vi "MOCVD_FrontPanel.vi"() -> ()   [LabVIEW 2011]
uses:
  low_level_proc/globals.vi
  editor_lib/Flow_Globals.vi
panel:
  out "Temp Actual":dbl caption="Actual (C)" format="%.2f"
  in  "Set":bool
  in  "Temp Setpoint":dbl caption="Setpoint (C)"
  in  "Heater":bool
  in  "Spinner":bool
  in  "Heater/Spinner Remote":bool caption="Remote"
  in  "Vac Remote":bool
  in  "Vac Exhaust":bool
  in  "Atm Exhaust":bool
  in  "Clear All Relays":bool
  in  "Stop":bool
  in  "?":T1(tab)
  in  "display N2 or H2":bool=TRUE
  in  "H2N2 Remote":bool caption="Remote"
  in  "N2 Target Flow":dbl caption="Target" min=0.0 max=1000.0
  in  "H2 Target Flow":dbl caption="Target" min=0.0 max=1000.0
  out "H2N2 Actual Flow":dbl caption="Actual"
  in  "N2 On":bool caption="On"
  in  "H2 On":bool caption="On"
  in  "Al Target Flow":dbl caption="Target" min=0.0 max=100.0 format="%.1f"
  out "Al Actual Flow":dbl caption="Actual" format="%.1f"
  in  "Al Remote":bool caption="Remote"
  in  "Al Active":bool caption="Active"
  in  "Al Bubbler In":bool caption="Bubbler In"
  in  "Al Run":bool caption="Run"
  out "Ga Flow2 label":string="Flow 2 (0-10 sscm)"
  out "Ga_Flow3_Label":string="Flow 3 (0-1000 sscm)" caption="String"
  out "Ga Actual Flow2":dbl caption="Actual" format="%.2f"
  out "Ga Actual Flow1":dbl caption="Actual" format="%.2f"
  out "Ga Actual Flow3":dbl caption="Actual"
  in  "Ga Target Flow 2":dbl caption="Target" min=0.0 max=10.0 format="%.2f"
  in  "Ga Target Flow 1":dbl caption="Target" min=0.0 max=1.0 format="%.2f"
  in  "Ga Active":bool caption="Active"
  in  "Ga Bubbler In":bool caption="Bubbler In"
  in  "Ga Run":bool caption="Run"
  in  "Ga H2 Dilute":bool caption="Dilute"
  in  "Ga Remote":bool caption="Remote"
  in  "Ga Target Flow 3":dbl caption="Target" min=0.0 max=1000.0
  in  "In Target Flow":dbl caption="Target" min=0.0 max=100.0 format="%.1f"
  out "In Actual Flow":dbl caption="Actual" format="%.1f"
  in  "In Remote":bool caption="Remote"
  in  "In Active":bool caption="Active"
  in  "In Bubbler In":bool caption="Bubbler In"
  in  "In Run":bool caption="Run"
  in  "P_gas Target Flow":dbl caption="Target" min=0.0 max=1000.0 format="%.1f"
  out "P Actual Flow":dbl caption="Actual" format="%.1f"
  in  "P gas Remote":bool caption="Remote"
  in  "P gas Active":bool caption="Active"
  in  "P Gas In":bool caption="Gas In"
  in  "P gas Run":bool caption="Run"
  in  "P gas H2 Purge":bool caption="H2 Purge"
  in  "AsH3 gas Target Flow":dbl caption="Target" min=0.0 max=1000.0 format="%.2f"
  out "As Actual Flow":dbl caption="Actual" format="%.2f"
  in  "As gas Run":bool caption="Run"
  in  "As gas H2 Purge":bool caption="H2 Purge"
  in  "As gas Active":bool caption="Active"
  in  "As Gas In":bool caption="Gas In"
  in  "As gas Remote":bool caption="Remote"
  in  "Pbub Target Flow":dbl caption="Target" min=0.0 max=100.0 format="%.1f"
  out "Pbub Actual Flow":dbl caption="Actual" format="%.1f"
  in  "Pbub Remote":bool caption="Remote"
  in  "Pbub Active":bool caption="Active"
  in  "Pbub Bubbler In":bool caption="Bubbler In"
  in  "Pbub Run":bool caption="Run"
  in  "ASL Target Flow":dbl caption="Target" min=0.0 max=100.0 format="%.1f"
  out "ASL Actual Flow":dbl caption="Actual" format="%.1f"
  in  "ASL Remote":bool caption="Remote"
  in  "ASL Active":bool caption="Active"
  in  "ASL Bubbler In":bool caption="Bubbler In"
  in  "ASL Run":bool caption="Run"
  in  "P or N":enum32{"P-Dopant", "N-Dopant"}(tab)
  out "Pdop flow 2 label":string="Flow 2 (0-100 sscm)"
  out "PDop Flow3 label":string="Flow 3 (0-1000 sscm)"
  in  "P_Dop H2 Dilute":bool caption="Dilute"
  in  "P_Dop Run":bool caption="Run"
  in  "P_Dop Bubbler":bool caption="Bubbler In"
  in  "P_Dop Active":bool caption="Active"
  in  "PDop Target Flow 1":dbl caption="Target:" min=0.0 max=100.0 format="%.1f"
  in  "PDop Target Flow  2":dbl caption="Target:" min=0.0 max=100.0 format="%.1f"
  in  "PDop Target Flow  3":dbl caption="Target:" min=0.0 max=1000.0 format="%.1f"
  in  "P_Dop Remote":bool caption="Remote"
  out "Ndop flow 2 label":string="Flow 2 (0-100 sscm)"
  out "Ndop Flow 3 label":string="Flow 3 (0-1000 sscm)"
  in  "Set N Dopant Flow Rate 1":dbl caption="Target" min=0.0 max=100.0 format="%.1f"
  in  "Set N Dopant Flow Rate 2":dbl caption="Target" min=0.0 max=100.0 format="%.1f"
  in  "Set N Dopant Flow Rate 3":dbl caption="Target" min=0.0 max=1000.0 format="%#.0f"
  in  "N_Dop Remote":bool caption="Remote"
  in  "N_Dop H2 Dilute":bool caption="Dilute"
  in  "N_Dop Run":bool caption="Run"
  in  "N_Dop Active":bool caption="Active"
  in  "N_Dop Bubbler":bool caption="Bubbler In"
  in  "6940B GPIB Address":string="23"
  # "Flow (0-1000 sccm)"
  # "N2"
  # "H2"
  # "N2"
  # "H2"
  # "Flow (0-100 sscm)"
  # "Flow 1 (0-10 sscm)"
  # "Flow (0-100 sscm)"
  # "Flow (0-100 sscm)"
  # "Flow (0-10 sscm)"
  # "Flow (0-100 sscm)"
  # "Flow (0-100 sscm)"
  # "Flow 1 (0-100 sscm)"
  # "Flow 1 (0-100 sscm)"
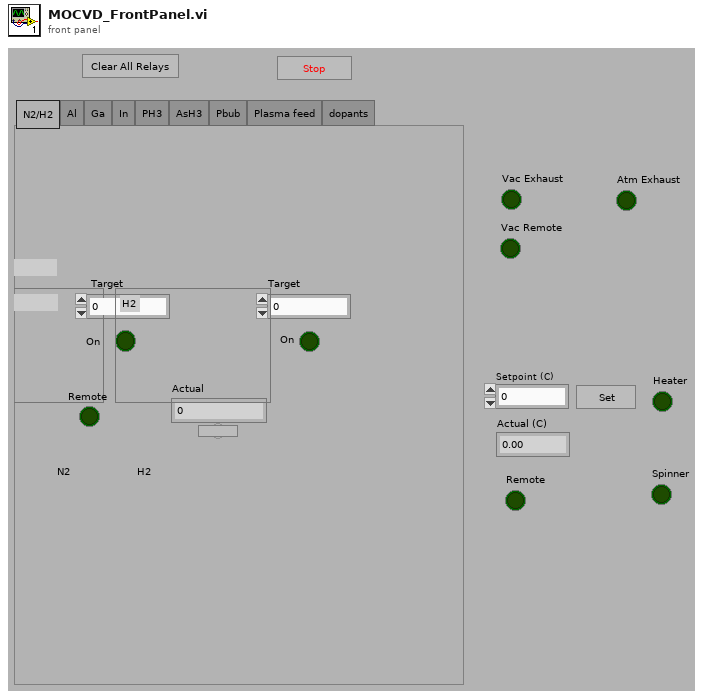
[diagram p1: front panel]
types:
  T1 = enum32{"N2/H2", "Al", "Ga", "In", "PH3", "AsH3", "Pbub", "Plasma feed", "dopants"}
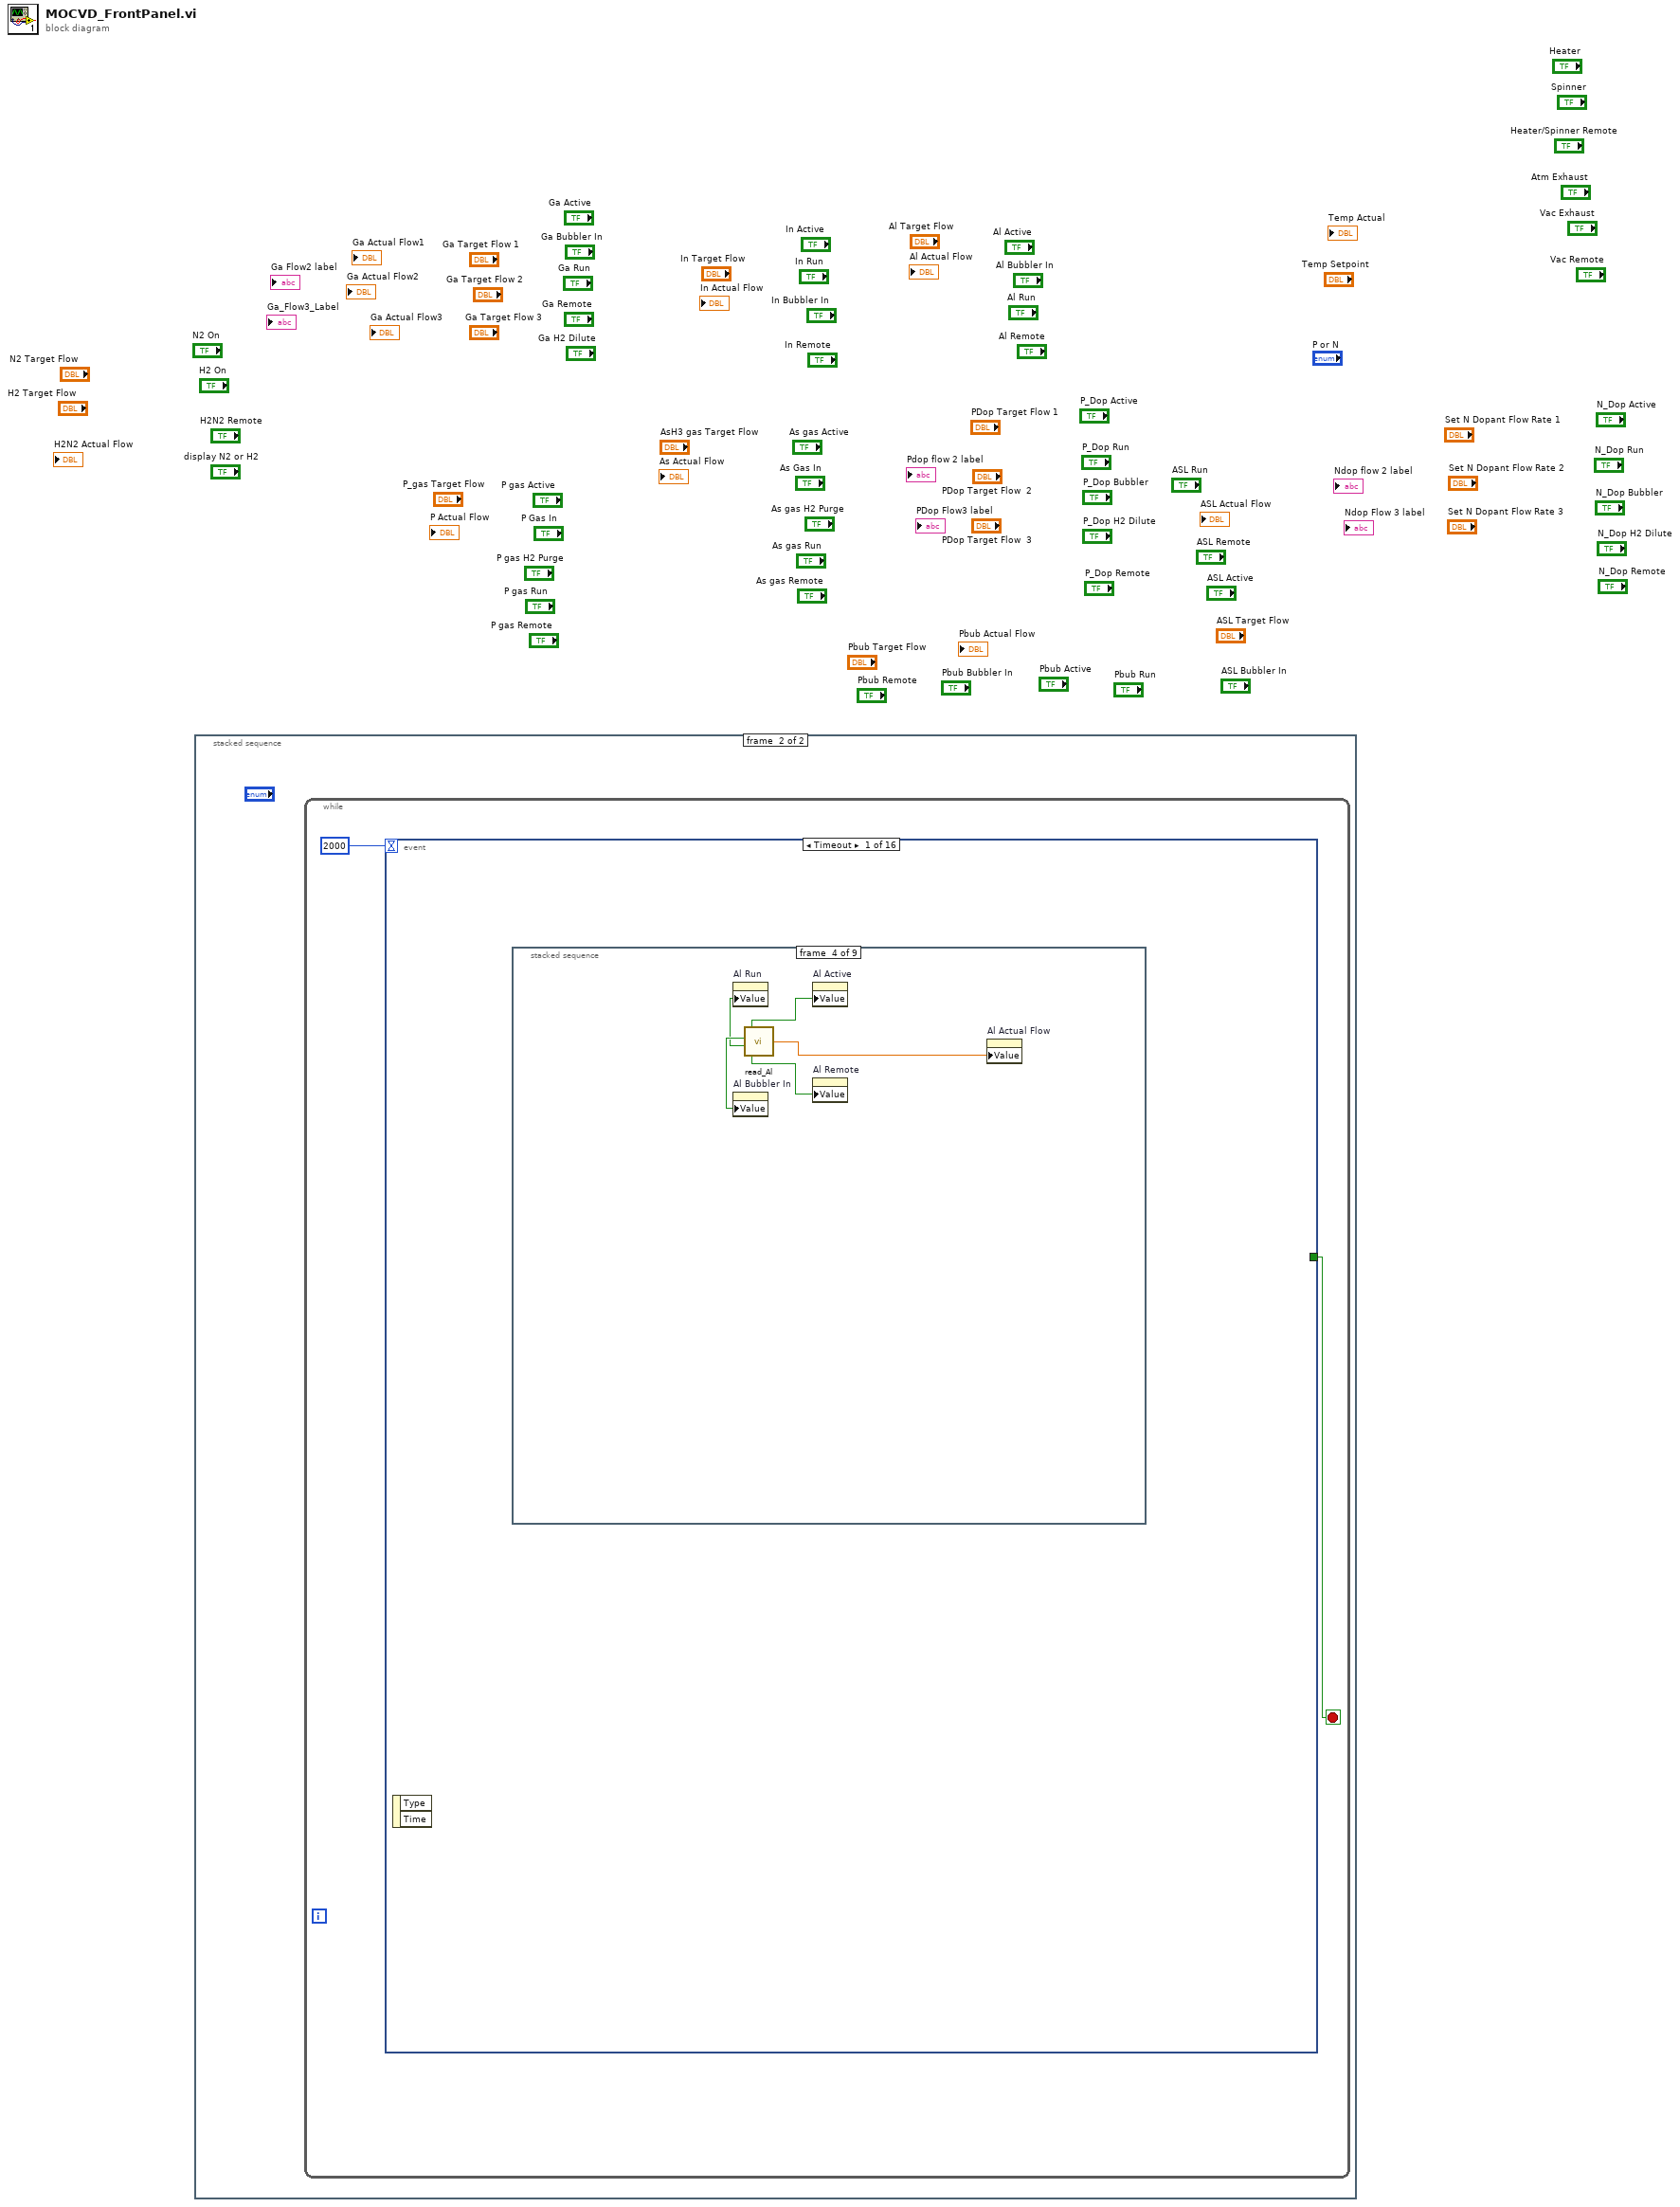
[diagram p0: block diagram]
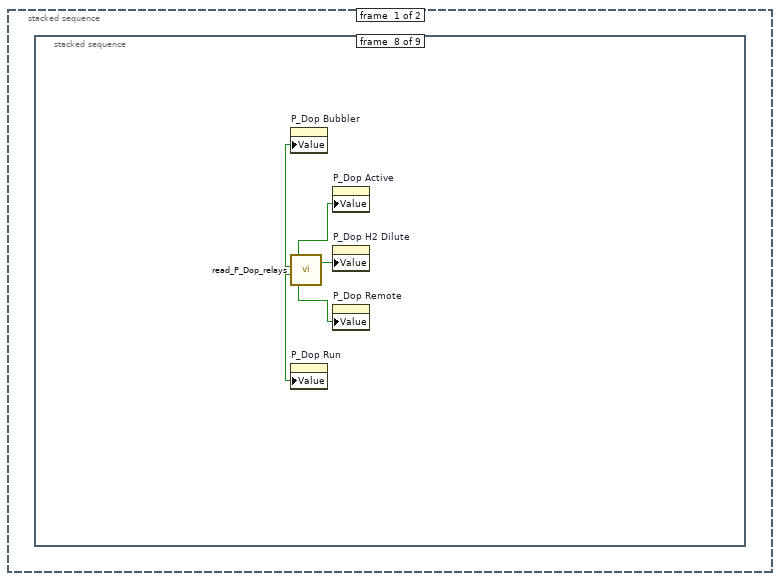
[diagram p2: hidden frame]
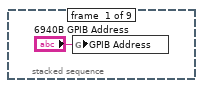
[diagram p3: hidden frame]
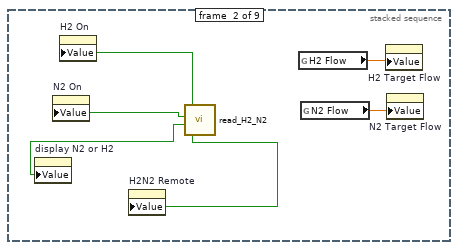
[diagram p4: hidden frame]
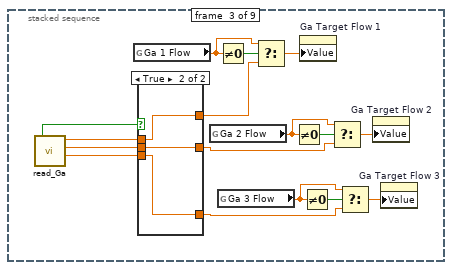
[diagram p5: hidden frame]
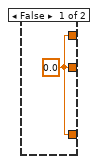
[diagram p6: hidden frame]
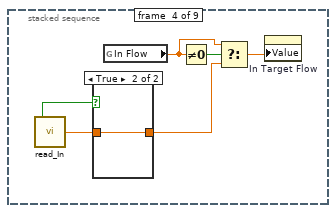
[diagram p7: hidden frame]
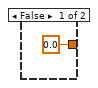
[diagram p8: hidden frame]
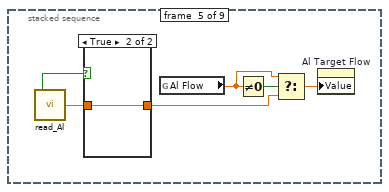
[diagram p9: hidden frame]
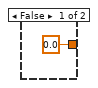
[diagram p10: hidden frame]
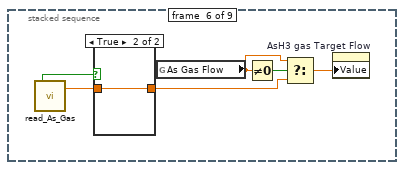
[diagram p11: hidden frame]
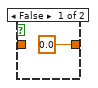
[diagram p12: hidden frame]
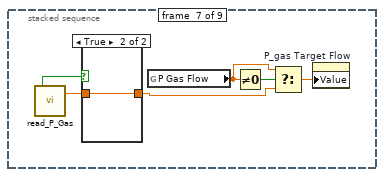
[diagram p13: hidden frame]
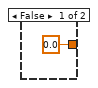
[diagram p14: hidden frame]
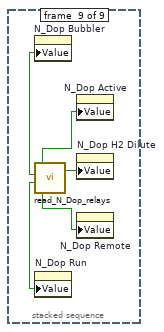
[diagram p15: hidden frame]
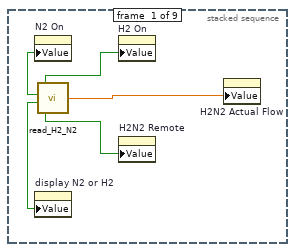
[diagram p16: hidden frame]
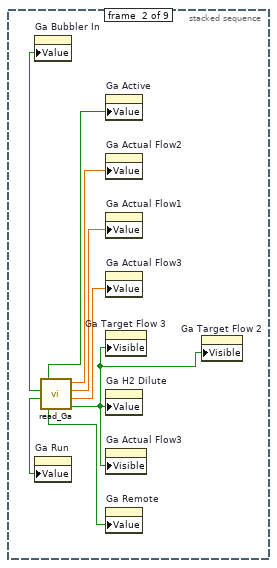
[diagram p17: hidden frame]
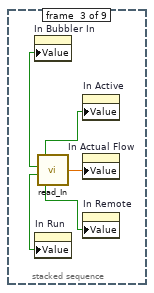
[diagram p18: hidden frame]
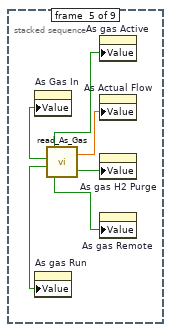
[diagram p19: hidden frame]
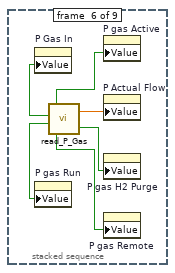
[diagram p20: hidden frame]
diagram:
  n1 = stacked-sequence {
    frame #0 {
      n2 = stacked-sequence {
        frame #0 {
          n3 = global write "globals.vi" "GPIB Address"("6940B GPIB Address") -> ()
        }
        frame #1 {
          n4 = call "read_H2_N2.vi"() -> ("Remote"=w5:bool, "Display H2N2"=w4:bool, "N2 Active"=w7:bool, "H2 Active"=w6:bool)  [unwired: 1 out]
          n5 = property on="display N2 or H2" class="Bool (strict)"("Value"=w4) -> ()  [unwired: 2 in, 2 out]
          n6 = property on="N2 On" class="Bool (strict)"("Value"=w7) -> ()  [unwired: 2 in, 2 out]
          n7 = property on="H2 On" class="Bool (strict)"("Value"=w6) -> ()  [unwired: 2 in, 2 out]
          n8 = property on="H2N2 Remote" class="Bool (strict)"("Value"=w5) -> ()  [unwired: 2 in, 2 out]
          n9 = global read "Flow_Globals.vi" "H2 Flow"() -> (w3:dbl)
          n10 = global read "Flow_Globals.vi" "N2 Flow"() -> (w2:dbl)
          n11 = property on="H2 Target Flow" class="DigNum (strict)"("Value"=w3) -> ()  [unwired: 2 in, 2 out]
          n12 = property on="N2 Target Flow" class="DigNum (strict)"("Value"=w2) -> ()  [unwired: 2 in, 2 out]
        }
        frame #2 {
          n13 = call "read_Ga.vi"() -> ("GAMFC3"=w22:dbl, "GAMFC2"=w23:dbl, "GAMFC1"=w21:dbl, "Active"=w20:bool)  [unwired: 4 out]
          n14 = global read "Flow_Globals.vi" "Ga 1 Flow"() -> (w18:dbl)
          n15 = case shown="True" w20 {
            tunnel: w23 -> [_ w26]
            tunnel: w22 -> [_ w25]
            tunnel: w21 -> [_ w27]
            tunnel: [w24 w27] -> w17
            tunnel: [w24 w26] -> w13
            tunnel: [w24 w25] -> w9
            frame False {
              w24 = 0.0 ("GAMFC2")
            }
            frame True {
            }
          }
          n16 = global read "Flow_Globals.vi" "Ga 2 Flow"() -> (w14:dbl)
          n17 = Not Equal To 0?(x=w18) -> (x != 0?=w19:bool)
          n18 = global read "Flow_Globals.vi" "Ga 3 Flow"() -> (w10:dbl)
          n19 = Select(t=w18, s=w19, f=w17) -> (s? t:f=w16:dbl)
          n20 = Not Equal To 0?(x=w14) -> (x != 0?=w15:bool)
          n21 = property on="Ga Target Flow 1" class="DigNum (strict)"("Value"=w16) -> ()  [unwired: 2 in, 2 out]
          n22 = Not Equal To 0?(x=w10) -> (x != 0?=w11:bool)
          n23 = Select(t=w14, s=w15, f=w13) -> (s? t:f=w12:dbl)
          n24 = Select(t=w10, s=w11, f=w9) -> (s? t:f=w8:dbl)
          n25 = property on="Ga Target Flow 2" class="DigNum (strict)"("Value"=w12) -> ()  [unwired: 2 in, 2 out]
          n26 = property on="Ga Target Flow 3" class="DigNum (strict)"("Value"=w8) -> ()  [unwired: 2 in, 2 out]
        }
        frame #3 {
          n27 = call "read_In.vi"() -> ("INMFC1"=w32:dbl, "Active"=w33:bool)  [unwired: 3 out]
          n28 = case shown="True" w33 {
            tunnel: [0.0 ("Actual In Flow Rate") w35] -> w29
            tunnel: w32 -> [_ w35]
            frame False {
            }
            frame True {
            }
          }
          n29 = global read "Flow_Globals.vi" "In Flow"() -> (w30:dbl)
          n30 = Not Equal To 0?(x=w30) -> (x != 0?=w31:bool)
          n31 = Select(t=w30, s=w31, f=w29) -> (s? t:f=w28:dbl)
          n32 = property on="In Target Flow" class="DigNum (strict)"("Value"=w28) -> ()  [unwired: 2 in, 2 out]
        }
        frame #4 {
          n33 = call "read_Al.vi"() -> ("ALMFC1"=w41:dbl, "Active"=w40:bool)  [unwired: 3 out]
          n34 = case shown="True" w40 {
            tunnel: [0.0 ("Actual Al Flow Rate") w43] -> w37
            tunnel: w41 -> [_ w43]
            frame False {
            }
            frame True {
            }
          }
          n35 = global read "Flow_Globals.vi" "Al Flow"() -> (w38:dbl)
          n36 = Not Equal To 0?(x=w38) -> (x != 0?=w39:bool)
          n37 = Select(t=w38, s=w39, f=w37) -> (s? t:f=w36:dbl)
          n38 = property on="Al Target Flow" class="DigNum (strict)"("Value"=w36) -> ()  [unwired: 2 in, 2 out]
        }
        frame #5 {
          n39 = call "read_As_Gas.vi"() -> ("As Gas Actual Flow Rate"=w48:dbl, "Active"=w49:bool)  [unwired: 4 out]
          n40 = case shown="True" w49 {
            tunnel: w48 -> [_ w51]
            tunnel: [0.0 ("As Gas Actual Flow Rate") w51] -> w45
            frame False {
            }
            frame True {
            }
          }
          n41 = global read "Flow_Globals.vi" "As Gas Flow"() -> (w46:dbl)
          n42 = Not Equal To 0?(x=w46) -> (x != 0?=w47:bool)
          n43 = Select(t=w46, s=w47, f=w45) -> (s? t:f=w44:dbl)
          n44 = property on="AsH3 gas Target Flow" class="DigNum (strict)"("Value"=w44) -> ()  [unwired: 2 in, 2 out]
        }
        frame #6 {
          n45 = call "read_P_Gas.vi"() -> ("P Gas Actual Flow Rate"=w56:dbl, "Active"=w57:bool)  [unwired: 4 out]
          n46 = case shown="True" w57 {
            tunnel: [0.0 ("P Gas Actual Flow Rate") w59] -> w53
            tunnel: w56 -> [_ w59]
            frame False {
            }
            frame True {
            }
          }
          n47 = global read "Flow_Globals.vi" "P Gas Flow"() -> (w54:dbl)
          n48 = Not Equal To 0?(x=w54) -> (x != 0?=w55:bool)
          n49 = Select(t=w54, s=w55, f=w53) -> (s? t:f=w52:dbl)
          n50 = property on="P_gas Target Flow" class="DigNum (strict)"("Value"=w52) -> ()  [unwired: 2 in, 2 out]
        }
        frame #7 {
          n51 = call "read_P_Dop_relays.vi"() -> ("P_Dop H2 Dilute"=w64:bool, "P_Dop Remote"=w61:bool, "P_Dop Run"=w62:bool, "P_Dop Bubbler"=w60:bool, "P_Dop Active"=w63:bool)  [unwired: 1 out]
          n52 = property on="P_Dop Bubbler" class="Bool (strict)"("Value"=w60) -> ()  [unwired: 2 in, 2 out]
          n53 = property on="P_Dop Run" class="Bool (strict)"("Value"=w62) -> ()  [unwired: 2 in, 2 out]
          n54 = property on="P_Dop Active" class="Bool (strict)"("Value"=w63) -> ()  [unwired: 2 in, 2 out]
          n55 = property on="P_Dop H2 Dilute" class="Bool (strict)"("Value"=w64) -> ()  [unwired: 2 in, 2 out]
          n56 = property on="P_Dop Remote" class="Bool (strict)"("Value"=w61) -> ()  [unwired: 2 in, 2 out]
        }
        frame #8 {
          n57 = call "read_N_Dop_relays.vi"() -> ("N_Dop H2 Dilute"=w69:bool, "N_Dop Remote"=w68:bool, "N_Dop Run"=w67:bool, "N_Dop Bubbler"=w66:bool, "N_Dop Active"=w65:bool)  [unwired: 1 out]
          n58 = property on="N_Dop Bubbler" class="Bool (strict)"("Value"=w66) -> ()  [unwired: 2 in, 2 out]
          n59 = property on="N_Dop Run" class="Bool (strict)"("Value"=w67) -> ()  [unwired: 2 in, 2 out]
          n60 = property on="N_Dop Active" class="Bool (strict)"("Value"=w65) -> ()  [unwired: 2 in, 2 out]
          n61 = property on="N_Dop H2 Dilute" class="Bool (strict)"("Value"=w69) -> ()  [unwired: 2 in, 2 out]
          n62 = property on="N_Dop Remote" class="Bool (strict)"("Value"=w68) -> ()  [unwired: 2 in, 2 out]
        }
      }
    }
    frame #1 {
      n63 = while {
        stop <- w71 stop-if-true
        n64 = event shown="[0] Timeout" {
          selector: _ -> [_ _ _ _ _ _ _ _ _ _ _ _ _ _ _ _]
          dyn-events: _ -> [_ _ _ _ _ _ _ _ _ _ _ _ _ _ _ _]
          timeout: 2000 -> [_ _ _ _ _ _ _ _ _ _ _ _ _ _ _ _]
          tunnel: [_ _ _ "Stop" _ _ _ _ _ _ _ _ _ _ _ _] -> w71
          event Timeout {
            n65 = event-data() -> ()  [unwired: 3 out]
            n66 = stacked-sequence {
              frame #0 {
                n67 = call "read_H2_N2.vi"() -> ("H2N2 Flow Rate"=w72:dbl, "Remote"=w76:bool, "Display H2N2"=w75:bool, "N2 Active"=w74:bool, "H2 Active"=w73:bool)
                n68 = property on="N2 On" class="Bool (strict)"("Value"=w74) -> ()  [unwired: 2 in, 2 out]
                n69 = property on="display N2 or H2" class="Bool (strict)"("Value"=w75) -> ()  [unwired: 2 in, 2 out]
                n70 = property on="H2 On" class="Bool (strict)"("Value"=w73) -> ()  [unwired: 2 in, 2 out]
                n71 = property on="H2N2 Remote" class="Bool (strict)"("Value"=w76) -> ()  [unwired: 2 in, 2 out]
                n72 = property on="H2N2 Actual Flow" class="DigNum (strict)"("Value"=w72) -> ()  [unwired: 2 in, 2 out]
              }
              frame #1 {
                n73 = call "read_Ga.vi"() -> ("H2 Dilute"=w77:bool, "GAMFC3"=w78:dbl, "GAMFC2"=w80:dbl, "GAMFC1"=w79:dbl, "Remote"=w83:bool, "Run"=w84:bool, "Bubbler In"=w81:bool, "Active"=w82:bool)
                n74 = property on="Ga Bubbler In" class="Bool (strict)"("Value"=w81) -> ()  [unwired: 2 in, 2 out]
                n75 = property on="Ga Run" class="Bool (strict)"("Value"=w84) -> ()  [unwired: 2 in, 2 out]
                n76 = property on="Ga Active" class="Bool (strict)"("Value"=w82) -> ()  [unwired: 2 in, 2 out]
                n77 = property on="Ga Actual Flow2" class="DigNum (strict)"("Value"=w79) -> ()  [unwired: 2 in, 2 out]
                n78 = property on="Ga Actual Flow1" class="DigNum (strict)"("Value"=w80) -> ()  [unwired: 2 in, 2 out]
                n79 = property on="Ga Actual Flow3" class="DigNum (strict)"("Value"=w78) -> ()  [unwired: 2 in, 2 out]
                n80 = property on="Ga Target Flow 3" class="DigNum (strict)"("Visible"=w77) -> ()  [unwired: 2 in, 2 out]
                n81 = property on="Ga H2 Dilute" class="Bool (strict)"("Value"=w77) -> ()  [unwired: 2 in, 2 out]
                n82 = property on="Ga Actual Flow3" class="DigNum (strict)"("Visible"=w77) -> ()  [unwired: 2 in, 2 out]
                n83 = property on="Ga Remote" class="Bool (strict)"("Value"=w83) -> ()  [unwired: 2 in, 2 out]
                n84 = property on="Ga Target Flow 2" class="DigNum (strict)"("Visible"=w77) -> ()  [unwired: 2 in, 2 out]
              }
              frame #2 {
                n85 = call "read_In.vi"() -> ("INMFC1"=w85:dbl, "Remote"=w87:bool, "Run"=w86:bool, "Bubbler In"=w88:bool, "Active"=w89:bool)
                n86 = property on="In Bubbler In" class="Bool (strict)"("Value"=w88) -> ()  [unwired: 2 in, 2 out]
                n87 = property on="In Run" class="Bool (strict)"("Value"=w86) -> ()  [unwired: 2 in, 2 out]
                n88 = property on="In Active" class="Bool (strict)"("Value"=w89) -> ()  [unwired: 2 in, 2 out]
                n89 = property on="In Actual Flow" class="DigNum (strict)"("Value"=w85) -> ()  [unwired: 2 in, 2 out]
                n90 = property on="In Remote" class="Bool (strict)"("Value"=w87) -> ()  [unwired: 2 in, 2 out]
              }
              frame #3 {
                n91 = call "read_Al.vi"() -> ("ALMFC1"=w90:dbl, "Remote"=w91:bool, "Run"=w92:bool, "Bubbler In"=w93:bool, "Active"=w94:bool)
                n92 = property on="Al Run" class="Bool (strict)"("Value"=w92) -> ()  [unwired: 2 in, 2 out]
                n93 = property on="Al Bubbler In" class="Bool (strict)"("Value"=w93) -> ()  [unwired: 2 in, 2 out]
                n94 = property on="Al Active" class="Bool (strict)"("Value"=w94) -> ()  [unwired: 2 in, 2 out]
                n95 = property on="Al Remote" class="Bool (strict)"("Value"=w91) -> ()  [unwired: 2 in, 2 out]
                n96 = property on="Al Actual Flow" class="DigNum (strict)"("Value"=w90) -> ()  [unwired: 2 in, 2 out]
              }
              frame #4 {
                n97 = call "read_As_Gas.vi"() -> ("H2 Flush"=w96:bool, "As Gas Actual Flow Rate"=w95:dbl, "Remote"=w100:bool, "Run"=w99:bool, "Gas In"=w98:bool, "Active"=w97:bool)
                n98 = property on="As Gas In" class="Bool (strict)"("Value"=w98) -> ()  [unwired: 2 in, 2 out]
                n99 = property on="As gas Run" class="Bool (strict)"("Value"=w99) -> ()  [unwired: 2 in, 2 out]
                n100 = property on="As gas Active" class="Bool (strict)"("Value"=w97) -> ()  [unwired: 2 in, 2 out]
                n101 = property on="As Actual Flow" class="DigNum (strict)"("Value"=w95) -> ()  [unwired: 2 in, 2 out]
                n102 = property on="As gas H2 Purge" class="Bool (strict)"("Value"=w96) -> ()  [unwired: 2 in, 2 out]
                n103 = property on="As gas Remote" class="Bool (strict)"("Value"=w100) -> ()  [unwired: 2 in, 2 out]
              }
              frame #5 {
                n104 = call "read_P_Gas.vi"() -> ("H2 Flush"=w102:bool, "P Gas Actual Flow Rate"=w101:dbl, "Remote"=w106:bool, "Run"=w105:bool, "Gas In"=w104:bool, "Active"=w103:bool)
                n105 = property on="P Gas In" class="Bool (strict)"("Value"=w104) -> ()  [unwired: 2 in, 2 out]
                n106 = property on="P gas Run" class="Bool (strict)"("Value"=w105) -> ()  [unwired: 2 in, 2 out]
                n107 = property on="P gas Active" class="Bool (strict)"("Value"=w103) -> ()  [unwired: 2 in, 2 out]
                n108 = property on="P Actual Flow" class="DigNum (strict)"("Value"=w101) -> ()  [unwired: 2 in, 2 out]
                n109 = property on="P gas H2 Purge" class="Bool (strict)"("Value"=w102) -> ()  [unwired: 2 in, 2 out]
                n110 = property on="P gas Remote" class="Bool (strict)"("Value"=w106) -> ()  [unwired: 2 in, 2 out]
              }
              frame #6 {
                n111 = call "read_vacuum.vi"() -> ("Vac Remote"=w109:bool, "Atm Exhaust"=w108:bool, "Vac Exhaust"=w107:bool)
                n112 = property on="Vac Exhaust" class="Bool (strict)"("Value"=w107) -> ()  [unwired: 2 in, 2 out]
                n113 = property on="Atm Exhaust" class="Bool (strict)"("Value"=w108) -> ()  [unwired: 2 in, 2 out]
                n114 = property on="Vac Remote" class="Bool (strict)"("Value"=w109) -> ()  [unwired: 2 in, 2 out]
              }
              frame #7 {
                n115 = call "read_heater_spinner.vi"() -> ("Heater/Spinner Remote"=w112:bool, "Spinner"=w111:bool, "Heater"=w110:bool)  [unwired: 7 out]
                n116 = property on="Spinner" class="Bool (strict)"("Value"=w111) -> ()  [unwired: 2 in, 2 out]
                n117 = property on="Heater/Spinner Remote" class="Bool (strict)"("Value"=w112) -> ()  [unwired: 2 in, 2 out]
                n118 = property on="Heater" class="Bool (strict)"("Value"=w110) -> ()  [unwired: 2 in, 2 out]
              }
              frame #8 {
                n119 = call "read_temp.vi"() -> ("Temperature (C)"=w113:dbl)  [unwired: 1 out]
                n120 = property on="Temp Actual" class="DigNum (strict)"("Value"=w113) -> ()  [unwired: 2 in, 2 out]
              }
            }
          }
          event "Set": Value Change {
            n121 = event-data() -> ()  [unwired: 6 out]
            n122 = property on="Temp Setpoint" class="DigNum (strict)"() -> ("Value"=w114:dbl)  [unwired: 2 in, 2 out]
            n123 = call "write_temp.vi"("Temperature (C)"=w114) -> ()  [unwired: 1 out]
          }
          event "Clear All Relays": Mouse Down {
            n124 = event-data() -> ()  [unwired: 8 out]
            n125 = flat-sequence {
              frame #0 {
                n126 = call "clear_all_relays.vi"() -> ()  [unwired: 2 out]
              }
              frame #1 {
                n127 = property on="Clear All Relays" class="Bool (strict)"("Value"=FALSE ("Clear All Relays")) -> ()  [unwired: 2 in, 2 out]
              }
            }
          }
          event "Stop": Value Change {
            n128 = event-data() -> ()  [unwired: 7 out]
          }
          event "H2N2 Remote", "display N2 or H2", "N2 On", "H2 On", "N2 Target Flow", "H2 Target Flow": Value Change {
            n129 = event-data() -> ()  [unwired: 7 out]
            n130 = property on="H2 On" class="Bool (strict)"() -> ("Value"=w118:bool)  [unwired: 2 in, 2 out]
            n131 = property on="H2 Target Flow" class="DigNum (strict)"() -> ("Value"=w121:dbl)  [unwired: 2 in, 2 out]
            n132 = property on="H2N2 Remote" class="Bool (strict)"() -> ("Value"=w117:bool)  [unwired: 2 in, 2 out]
            n133 = property on="N2 Target Flow" class="DigNum (strict)"() -> ("Value"=w120:dbl)  [unwired: 2 in, 2 out]
            n134 = property on="N2 On" class="Bool (strict)"() -> ("Value"=w119:bool)  [unwired: 2 in, 2 out]
            n135 = property on="display N2 or H2" class="Bool (strict)"() -> ("Value"=w122:bool)  [unwired: 2 in, 2 out]
            n136 = call "set_H2N2_display.vi"("Manifold N2 Flow"=w120, "Manifold H2 Flow"=w121, "Display H2 or N2"=w122, "H2 Active"=w118, "N2 Active"=w119, "Remote"=w117) -> ()
          }
          event "In Remote", "In Active", "In Bubbler In", "In Run", "In Target Flow": Value Change {
            n137 = event-data() -> ()  [unwired: 7 out]
            n138 = property on="In Target Flow" class="DigNum (strict)"() -> ("Value"=w127:dbl)  [unwired: 2 in, 2 out]
            n139 = property on="In Bubbler In" class="Bool (strict)"() -> ("Value"=w123:bool)  [unwired: 2 in, 2 out]
            n140 = property on="In Run" class="Bool (strict)"() -> ("Value"=w125:bool)  [unwired: 2 in, 2 out]
            n141 = property on="In Active" class="Bool (strict)"() -> ("Value"=w124:bool)  [unwired: 2 in, 2 out]
            n142 = property on="In Remote" class="Bool (strict)"() -> ("Value"=w126:bool)  [unwired: 2 in, 2 out]
            n143 = call "set_In.vi"("INMFC1"=w127, "Remote"=w126, "Run"=w125, "Bubbler In"=w123, "Active"=w124) -> ()  [unwired: 5 in]
          }
          event "Pbub Remote", "Pbub Active", "Pbub Bubbler In", "Pbub Run", "Pbub Target Flow": Value Change {
            n144 = event-data() -> ()  [unwired: 7 out]
            n145 = property on="Pbub Target Flow" class="DigNum (strict)"() -> ("Value"=w132:dbl)  [unwired: 2 in, 2 out]
            n146 = property on="Pbub Run" class="Bool (strict)"() -> ("Value"=w129:bool)  [unwired: 2 in, 2 out]
            n147 = property on="Pbub Bubbler In" class="Bool (strict)"() -> ("Value"=w130:bool)  [unwired: 2 in, 2 out]
            n148 = property on="Pbub Active" class="Bool (strict)"() -> ("Value"=w131:bool)  [unwired: 2 in, 2 out]
            n149 = property on="Pbub Remote" class="Bool (strict)"() -> ("Value"=w128:bool)  [unwired: 2 in, 2 out]
            n150 = call "set_P_Liq.vi"("flow 1"=w132, "Remote"=w128, "Run"=w129, "Bubbler In"=w130, "Active"=w131) -> ()  [unwired: 5 in]
          }
          event "ASL Target Flow", "ASL Active", "ASL Bubbler In", "ASL Run", "ASL Remote": Value Change {
            n151 = event-data() -> ()  [unwired: 7 out]
            n152 = property on="ASL Active" class="Bool (strict)"() -> ("Value"=w136:bool)  [unwired: 2 in, 2 out]
            n153 = property on="ASL Bubbler In" class="Bool (strict)"() -> ("Value"=w135:bool)  [unwired: 2 in, 2 out]
            n154 = property on="ASL Run" class="Bool (strict)"() -> ("Value"=w134:bool)  [unwired: 2 in, 2 out]
            n155 = property on="ASL Target Flow" class="DigNum (strict)"() -> ("Value"=w137:dbl)  [unwired: 2 in, 2 out]
            n156 = property on="ASL Remote" class="Bool (strict)"() -> ("Value"=w133:bool)  [unwired: 2 in, 2 out]
            n157 = call "set_As_Liq.vi"("ASLMFC1"=w137, "Remote"=w133, "Run"=w134, "Bubbler In"=w135, "Active"=w136) -> ()  [unwired: 5 in]
          }
          event "Al Remote", "Al Active", "Al Bubbler In", "Al Run", "Al Target Flow": Value Change {
            n158 = event-data() -> ()  [unwired: 7 out]
            n159 = property on="Al Target Flow" class="DigNum (strict)"() -> ("Value"=w142:dbl)  [unwired: 2 in, 2 out]
            n160 = property on="Al Bubbler In" class="Bool (strict)"() -> ("Value"=w140:bool)  [unwired: 2 in, 2 out]
            n161 = property on="Al Active" class="Bool (strict)"() -> ("Value"=w141:bool)  [unwired: 2 in, 2 out]
            n162 = property on="Al Run" class="Bool (strict)"() -> ("Value"=w139:bool)  [unwired: 2 in, 2 out]
            n163 = property on="Al Remote" class="Bool (strict)"() -> ("Value"=w138:bool)  [unwired: 2 in, 2 out]
            n164 = call "set_Al.vi"("ALMFC1"=w142, "Remote"=w138, "Run"=w139, "Bubbler In"=w140, "Active"=w141) -> ()  [unwired: 5 out]
          }
          event "P gas Remote", "P gas Active", "P Gas In", "P gas Run", "P gas H2 Purge", "P_gas Target Flow": Value Change {
            n165 = event-data() -> ()  [unwired: 7 out]
            n166 = property on="P_gas Target Flow" class="DigNum (strict)"() -> ("Value"=w148:dbl)  [unwired: 2 in, 2 out]
            n167 = property on="P gas Active" class="Bool (strict)"() -> ("Value"=w147:bool)  [unwired: 2 in, 2 out]
            n168 = property on="P Gas In" class="Bool (strict)"() -> ("Value"=w146:bool)  [unwired: 2 in, 2 out]
            n169 = property on="P gas H2 Purge" class="Bool (strict)"() -> ("Value"=w145:bool)  [unwired: 2 in, 2 out]
            n170 = property on="P gas Run" class="Bool (strict)"() -> ("Value"=w144:bool)  [unwired: 2 in, 2 out]
            n171 = property on="P gas Remote" class="Bool (strict)"() -> ("Value"=w143:bool)  [unwired: 2 in, 2 out]
            n172 = call "set_P_gas.vi"("Run"=w144, "Gas In"=w146, "Active"=w147, "P_Gas Remote"=w143, "H2 Flush"=w145, "P_Gas Flow"=w148) -> ()
          }
          event "As gas Remote", "As gas Run", "As gas H2 Purge", "As Gas In", "As gas Active", "AsH3 gas Target Flow": Value Change {
            n173 = event-data() -> ()  [unwired: 7 out]
            n174 = property on="AsH3 gas Target Flow" class="DigNum (strict)"() -> ("Value"=w154:dbl)  [unwired: 2 in, 2 out]
            n175 = property on="As gas Active" class="Bool (strict)"() -> ("Value"=w153:bool)  [unwired: 2 in, 2 out]
            n176 = property on="As Gas In" class="Bool (strict)"() -> ("Value"=w152:bool)  [unwired: 2 in, 2 out]
            n177 = property on="As gas H2 Purge" class="Bool (strict)"() -> ("Value"=w151:bool)  [unwired: 2 in, 2 out]
            n178 = property on="As gas Run" class="Bool (strict)"() -> ("Value"=w150:bool)  [unwired: 2 in, 2 out]
            n179 = property on="As gas Remote" class="Bool (strict)"() -> ("Value"=w149:bool)  [unwired: 2 in, 2 out]
            n180 = call "set_As_gas.vi"("Active"=w153, "As_Gas Flow"=w154, "Gas In"=w152, "H2 Flush"=w151, "Run"=w150, "Remote"=w149) -> ()  [unwired: 10 out]
          }
          event "Ga Active", "Ga Bubbler In", "Ga Run", "Ga Target Flow 1", "Ga Target Flow 2", "Ga Target Flow 3", "Ga Remote", "Ga H2 Dilute": Value Change {
            n181 = event-data() -> ()  [unwired: 6 out]
            n182 = property on="Ga Bubbler In" class="Bool (strict)"() -> ("Value"=w159:bool)  [unwired: 2 in, 2 out]
            n183 = property on="Ga Target Flow 1" class="DigNum (strict)"() -> ("Value"=w162:dbl)  [unwired: 2 in, 2 out]
            n184 = property on="Ga Target Flow 2" class="DigNum (strict)"() -> ("Value"=w161:dbl)  [unwired: 2 in, 2 out]
            n185 = property on="Ga Target Flow 3" class="DigNum (strict)"() -> ("Value"=w160:dbl)  [unwired: 2 in, 2 out]
            n186 = property on="Ga Active" class="Bool (strict)"() -> ("Value"=w158:bool)  [unwired: 2 in, 2 out]
            n187 = property on="Ga Run" class="Bool (strict)"() -> ("Value"=w156:bool)  [unwired: 2 in, 2 out]
            n188 = property on="Ga Remote" class="Bool (strict)"() -> ("Value"=w157:bool)  [unwired: 2 in, 2 out]
            n189 = property on="Ga H2 Dilute" class="Bool (strict)"() -> ("Value"=w155:bool)  [unwired: 2 in, 2 out]
            n190 = call "set_Ga.vi"("Active"=w158, "GAMFC3"=w160, "GAMFC2"=w161, "GAMFC1"=w162, "Bubbler In"=w159, "H2 Dilute"=w155, "Run"=w156, "Remote"=w157) -> ()  [unwired: 8 out]
            n191 = property on="Ga Actual Flow3" class="DigNum (strict)"("Visible"=w155) -> ()  [unwired: 2 in, 2 out]
            n192 = property on="Ga Target Flow 2" class="DigNum (strict)"("Visible"=w155) -> ()  [unwired: 2 in, 2 out]
            n193 = property on="Ga Target Flow 3" class="DigNum (strict)"("Visible"=w155) -> ()  [unwired: 2 in, 2 out]
            n194 = property on="Ga_Flow3_Label" class="Str"("Visible"=w155) -> ()  [unwired: 2 in, 2 out]
          }
          event "P_Dop Run", "P_Dop Bubbler", "P_Dop Active", "PDop Target Flow 1", "PDop Target Flow  2", "PDop Target Flow  3", "P_Dop Remote", "P_Dop H2 Dilute": Value Change {
            n195 = event-data() -> ()  [unwired: 7 out]
            n196 = property on="PDop Target Flow 1" class="DigNum (strict)"() -> ("Value"=w166:dbl)  [unwired: 2 in, 2 out]
            n197 = property on="PDop Target Flow  2" class="DigNum (strict)"() -> ("Value"=w165:dbl)  [unwired: 2 in, 2 out]
            n198 = property on="PDop Target Flow  3" class="DigNum (strict)"() -> ("Value"=w164:dbl)  [unwired: 2 in, 2 out]
            n199 = property on="P_Dop Active" class="Bool (strict)"() -> ("Value"=w169:bool)  [unwired: 2 in, 2 out]
            n200 = property on="P_Dop Bubbler" class="Bool (strict)"() -> ("Value"=w168:bool)  [unwired: 2 in, 2 out]
            n201 = property on="P_Dop Run" class="Bool (strict)"() -> ("Value"=w170:bool)  [unwired: 2 in, 2 out]
            n202 = property on="P_Dop Remote" class="Bool (strict)"() -> ("Value"=w171:bool)  [unwired: 2 in, 2 out]
            n203 = property on="P_Dop H2 Dilute" class="Bool (strict)"() -> ("Value"=w163:bool)  [unwired: 2 in, 2 out]
            n204 = call "set_P_Dop.vi"("P_Dop Active"=w169, "P_Dop Bubbler"=w168, "P_Dop H2 Dilute"=w163, "P_Dop Gas Source"=FALSE, "P_Dop Run"=w170, "P_Dop Remote"=w171, "P_Dop Flow 3"=w164, "P_Dop Flow 2"=w165, "P_Dop Flow 1"=w166) -> ()  [unwired: 1 in, 10 out]
            n205 = property on="Pdop flow 2 label" class="Str"("Visible"=w163) -> ()  [unwired: 2 in, 2 out]
            n206 = property on="PDop Target Flow  2" class="DigNum (strict)"("Visible"=w163) -> ()  [unwired: 2 in, 2 out]
            n207 = property on="PDop Target Flow  3" class="DigNum (strict)"("Visible"=w163) -> ()  [unwired: 2 in, 2 out]
            n208 = property on="PDop Flow3 label" class="Str"("Visible"=w163) -> ()  [unwired: 2 in, 2 out]
          }
          event "Set N Dopant Flow Rate 1", "Set N Dopant Flow Rate 2", "Set N Dopant Flow Rate 3", "N_Dop Remote", "N_Dop H2 Dilute", "N_Dop Run", "N_Dop Active", "N_Dop Bubbler": Value Change {
            n209 = event-data() -> ()  [unwired: 7 out]
            n210 = property on="N_Dop H2 Dilute" class="Bool (strict)"() -> ("Value"=w172:bool)  [unwired: 2 in, 2 out]
            n211 = property on="Set N Dopant Flow Rate 2" class="DigNum (strict)"("Visible"=w172) -> ()  [unwired: 2 in, 2 out]
            n212 = property on="Ndop flow 2 label" class="Str"("Visible"=w172) -> ()  [unwired: 2 in, 2 out]
            n213 = property on="Ndop Flow 3 label" class="Str"("Visible"=w172) -> ()  [unwired: 2 in, 2 out]
            n214 = property on="Set N Dopant Flow Rate 3" class="DigNum (strict)"("Visible"=w172) -> ()  [unwired: 2 in, 2 out]
            n215 = property on="N_Dop_Target_Flow_1" class="DigNum (strict)"() -> ("Value"=w175:dbl)  [unwired: 2 in, 2 out]
            n216 = property on="N_Dop_Target_Flow_2" class="DigNum (strict)"() -> ("Value"=w174:dbl)  [unwired: 2 in, 2 out]
            n217 = property on="N_Dop_Target_Flow_3" class="DigNum (strict)"() -> ("Value"=w173:dbl)  [unwired: 2 in, 2 out]
            n218 = property on="N_Dop Active" class="Bool (strict)"() -> ("Value"=w177:bool)  [unwired: 2 in, 2 out]
            n219 = property on="N_Dop Bubbler" class="Bool (strict)"() -> ("Value"=w179:bool)  [unwired: 2 in, 2 out]
            n220 = property on="N_Dop Run" class="Bool (strict)"() -> ("Value"=w178:bool)  [unwired: 2 in, 2 out]
            n221 = property on="N_Dop Remote" class="Bool (strict)"() -> ("Value"=w180:bool)  [unwired: 2 in, 2 out]
            n222 = call "set_N_Dop.vi"("Active"=w177, "Bubbler In"=w179, "H2 Dilute"=w172, "Gas Source In"=FALSE ("N_Dop Gas Source"), "Run"=w178, "Remote"=w180, "Flow 3"=w173, "Flow 2"=w174, "Flow 1"=w175) -> ()  [unwired: 1 in, 10 out]
          }
          event "Heater", "Spinner", "Heater/Spinner Remote": Value Change {
            n223 = event-data() -> ()  [unwired: 7 out]
            n224 = property on="Spinner" class="Bool (strict)"() -> ("Value"=w181:bool)  [unwired: 2 in, 2 out]
            n225 = property on="Heater/Spinner Remote" class="Bool (strict)"() -> ("Value"=w183:bool)  [unwired: 2 in, 2 out]
            n226 = property on="Heater" class="Bool (strict)"() -> ("Value"=w182:bool)  [unwired: 2 in, 2 out]
            n227 = call "set_heater_spinner.vi"("Remote"=w183, "Spinner"=w181, "Heater"=w182) -> ()  [unwired: 7 out]
          }
          event "Vac Remote", "Vac Exhaust", "Atm Exhaust": Value Change {
            n228 = event-data() -> ()  [unwired: 7 out]
            n229 = property on="Vac Remote" class="Bool (strict)"() -> ("Value"=w186:bool)  [unwired: 2 in, 2 out]
            n230 = property on="Vac Exhaust" class="Bool (strict)"() -> ("Value"=w185:bool)  [unwired: 2 in, 2 out]
            n231 = property on="Atm Exhaust" class="Bool (strict)"() -> ("Value"=w184:bool)  [unwired: 2 in, 2 out]
            n232 = call "set_vacuum.vi"("Remote"=w186, "Atm"=w184, "Vac Exhaust"=w185) -> ()
          }
        }
      }
    }
  }
